vi "Logging Slope.vi"(8 "error in (no error)":errorcluster, 11 "Heart Rate Params":T1) -> (0 "error out":errorcluster, 2 "appended array":dbl[](array[numeric]), 3 "Heart Rate Params Out":T1 caption="Heart Rate Params")   [LabVIEW 2017]
uses:
  Custom Controls/Heart Rate Parameters.ctl
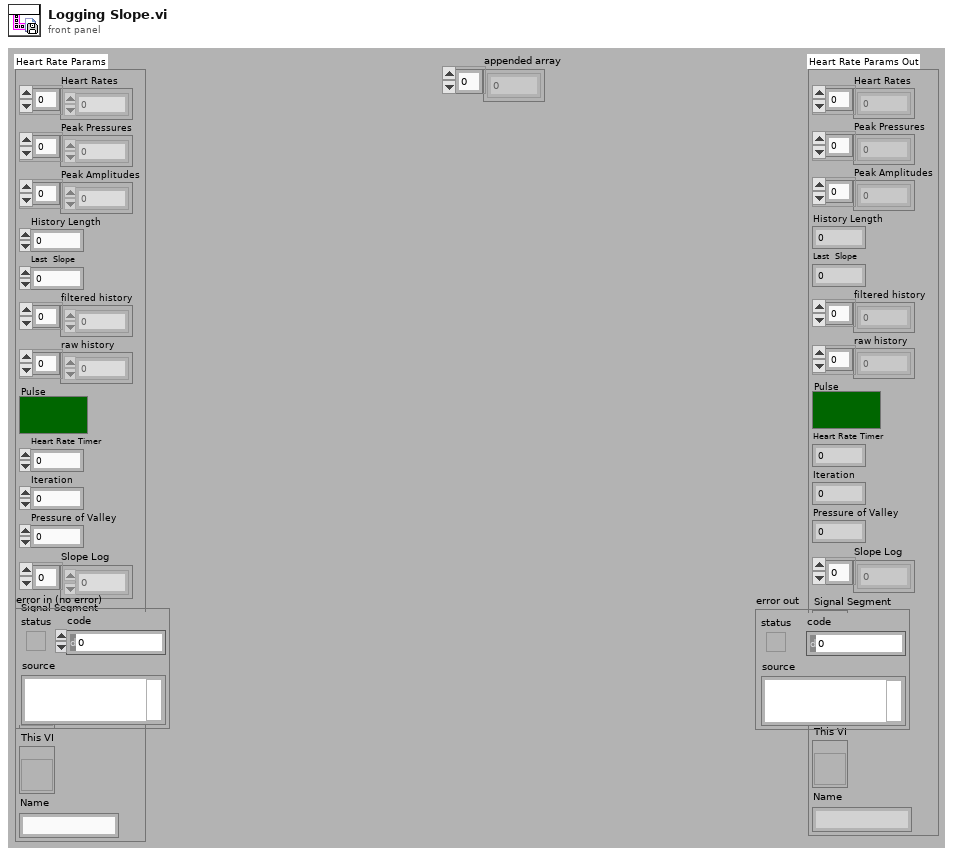
[diagram p1: front panel]
types:
  T1 = typedef "Heart Rate Parameters.ctl" = cluster{"Heart Rates":dbl[], "Peak Pressures":dbl[], "Peak Amplitudes":dbl[], "History Length":i32, "Last  Slope":dbl, "filtered history":dbl[], "raw history":dbl[], "Pulse":bool, "Heart Rate Timer":i32, "Iteration":u32, "Pressure of Valley":dbl, "Slope Log":dbl[], "Signal Segment":refnum<vi>, "Acquisition Graph":refnum<vi>, "This VI":refnum<vi>, "Name":string}
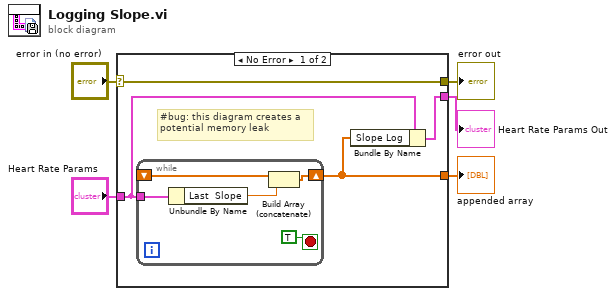
[diagram p0: block diagram]
diagram:
  n1 = case shown="No Error" "error in (no error)" {
    selector: "error in (no error)" -> [w9 w16]
    tunnel: [w7 _] -> w5
    tunnel: "Heart Rate Params" -> [w8 w15]
    tunnel: [w9 w16] -> w2
    tunnel: [w6 w15] -> w1
    frame No Error {
      # "#bug: this diagram creates a \npotential memory leak"
      n2 = while {
        tunnel: w8 -> [w14]
        shift-right: [w13] -> w7
        shift-left: _ -> [w12]
        stop <- TRUE stop-if-true
        n3 = Unbundle By Name(w14) -> ("Last  Slope"=w10:dbl)
        n4 = Build Array (concatenate)(w12, w10) -> (w13:dbl[])
      }
      n5 = Bundle By Name(cluster=w8, "Slope Log"=w7) -> (w6:T1)
    }
    frame Error {
    }
  }
  "Heart Rate Params Out" <- w1
  "appended array" <- w5
  "error out" <- w2
